vi "set_bit.vi"(1 "State":bool, 2 "Position":u16, 3 "Array":u8[](array[numeric])) -> (0 "Array 2":u8[](array[numeric]))   [LabVIEW 2022 SP3]
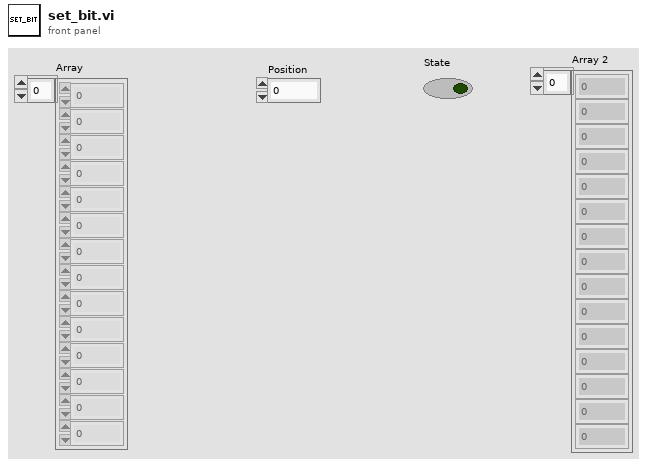
[diagram p1: front panel]
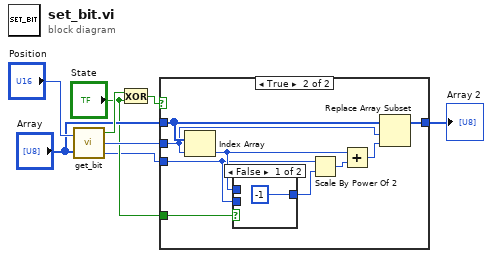
[diagram p0: block diagram]
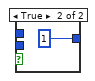
[diagram p3: hidden frame]
diagram:
  n1 = call "get_bit.vi"("Position"="Position", "INFO"="Array") -> ("Bit_Value"=w6:bool, "Byte_index"=w4:u16, "Bit_index"=w2:u16)
  n2 = Exclusive Or(1:"State", 2:w6) -> (0:w8:bool)
  n3 = case shown="True" w8 {
    tunnel: "Array" -> [w9 w15]
    tunnel: w4 -> [_ w14]
    tunnel: "State" -> [_ w18]
    tunnel: w2 -> [_ w16]
    tunnel: [w9 w13] -> w1
    frame False {
    }
    frame True {
      n4 = Index Array(array=w15, index=w14) -> (element=w17:u8)
      n5 = case shown="False" w18 {
        tunnel: w17 -> [_ _]
        tunnel: w16 -> [_ _]
        tunnel: [-1 u16 1 ("x")] -> w11
        frame False {
        }
        frame True {
        }
      }
      n6 = Scale By Power Of 2(n=w16, x=w11) -> (x*2^n=w12:i32)
      n7 = Add(x=w17, y=w12) -> (x+y=w10:i32)
      n8 = Replace Array Subset(array=w15, new element=w10, index=w14) -> (w13:u8[])
    }
  }
  "Array 2" <- w1
